vi "calc_VoltageRampWaveform_v0.03.vi"(0 "New input cluster":T1={"Which Position to use for Experiment"=enum."Jumper Safe Position", "Duration (s)"=0.0, "Delay (s)"=0.0, "Ramp Slope (mV/s)"=0.0, "Voltage Start (mV)"=1.0, "Replicates"=1.0, "Voltage End (mV)"=1.0, "Ramp Duration (s)"=0.0, "Vholding (mV)"=0.0, "Valve 1 Position"=2, "Valve 2 Position"=2, "Valve 3 Position"=2, "valve 1 used now?"=TRUE, "valve 2 used now?"=FALSE, "valve 3 used now? "=FALSE, "Maintain Final Voltage until end?"=TRUE, "protocol Preview"=[]} {"Valve 3 Position" min=1 max=8; "Valve 2 Position" min=1 max=8}, 1 "Clear Waveform?":bool, 5 "Old input cluster":T1={"Which Position to use for Experiment"=enum."Jumper Safe Position", "Duration (s)"=0.0, "Delay (s)"=0.0, "Ramp Slope (mV/s)"=0.0, "Voltage Start (mV)"=1.0, "Replicates"=1.0, "Voltage End (mV)"=1.0, "Ramp Duration (s)"=0.0, "Vholding (mV)"=0.0, "Valve 1 Position"=2, "Valve 2 Position"=2, "Valve 3 Position"=2, "valve 1 used now?"=TRUE, "valve 2 used now?"=FALSE, "valve 3 used now? "=FALSE, "Maintain Final Voltage until end?"=TRUE, "protocol Preview"=[]} {"Valve 3 Position" min=1 max=8; "Valve 2 Position" min=1 max=8}, 7 "sample freq":i32=10000, 11 "error in":errorcluster) -> (4 "output cluster":T1={"Which Position to use for Experiment"=enum."Jumper Safe Position", "Duration (s)"=0.0, "Delay (s)"=0.0, "Ramp Slope (mV/s)"=0.0, "Voltage Start (mV)"=1.0, "Replicates"=1.0, "Voltage End (mV)"=1.0, "Ramp Duration (s)"=0.0, "Vholding (mV)"=0.0, "Valve 1 Position"=2, "Valve 2 Position"=2, "Valve 3 Position"=2, "valve 1 used now?"=TRUE, "valve 2 used now?"=FALSE, "valve 3 used now? "=FALSE, "Maintain Final Voltage until end?"=TRUE, "protocol Preview"=[]} {"Valve 3 Position" min=1 max=8; "Valve 2 Position" min=1 max=8}, 15 "error out":errorcluster)   [LabVIEW 2019]
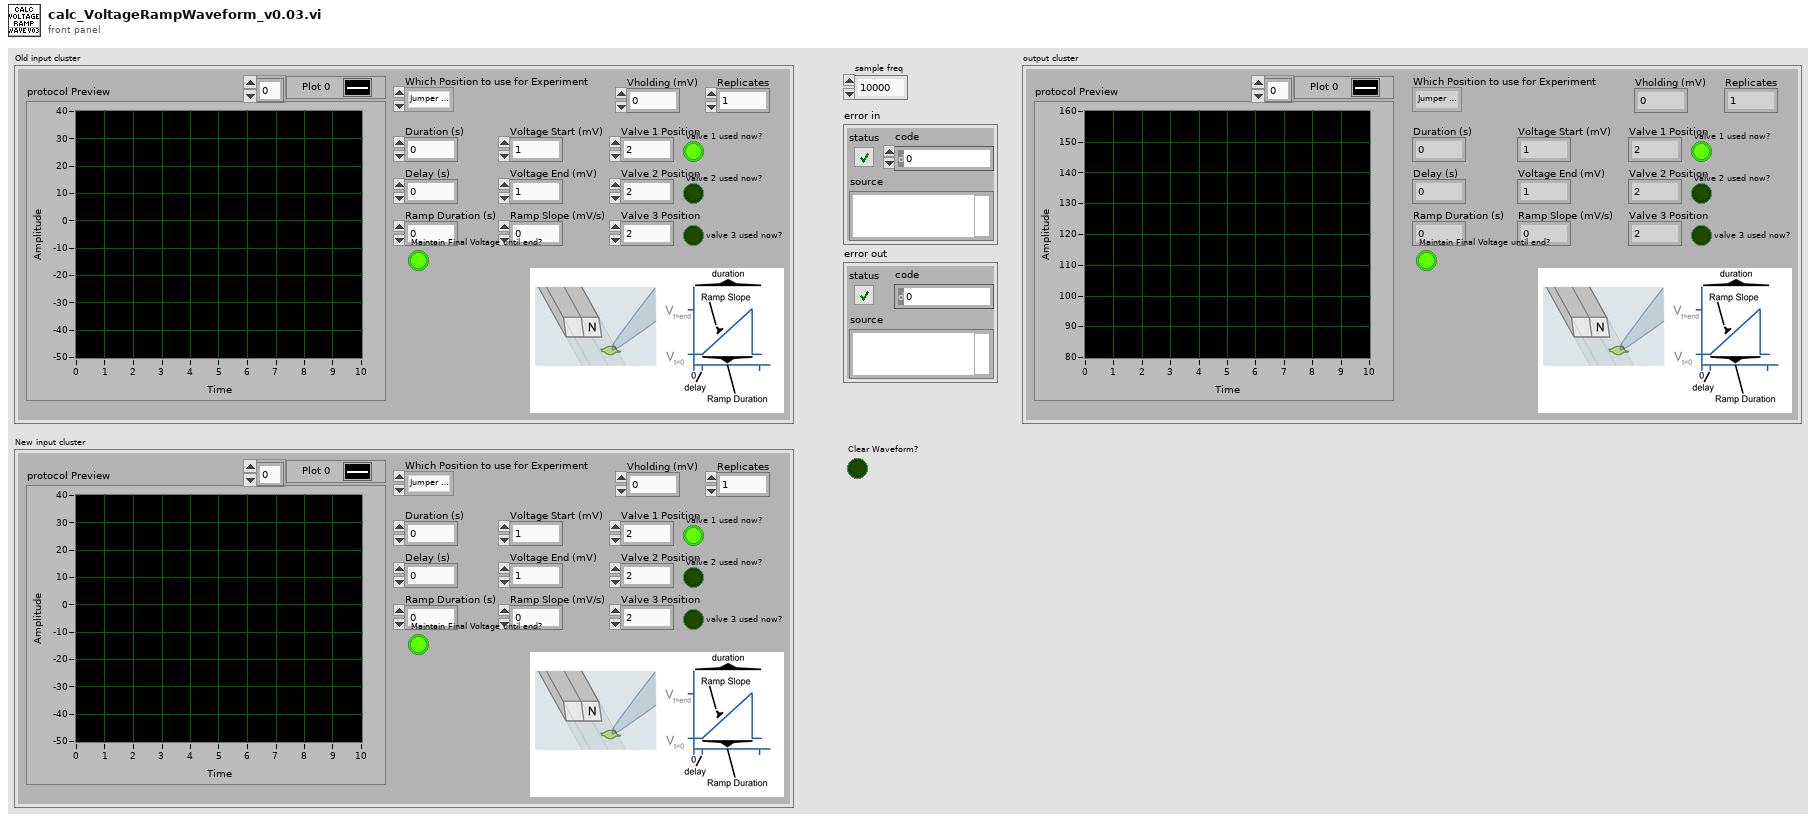
[diagram p1: front panel]
types:
  T1 = cluster{"Which Position to use for Experiment":enum16{"Jumper Safe Position", "Experiment Safe Position", "Jumper Position A", "Jumper Position B", "Jumper Position C", "Jumper Position o-A", "Jumper Position A-o", "Jumper Position A-B", "Jumper Position B-A", "Jumper Position B-C", "Jumper Position C-B", "Jumper Position C-o", "Jumper Position o-C", "Don't Move"}, "Duration (s)":dbl, "Delay (s)":dbl, "Ramp Slope (mV/s)":dbl, "Voltage Start (mV)":dbl, "Replicates":dbl, "Voltage End (mV)":dbl, "Ramp Duration (s)":dbl, "Vholding (mV)":dbl, "Valve 1 Position":i16, "Valve 2 Position":i16, "Valve 3 Position":i16, "valve 1 used now?":bool, "valve 2 used now?":bool, "valve 3 used now? ":bool, "Maintain Final Voltage until end?":bool, "protocol Preview":waveform(dbl)[]}
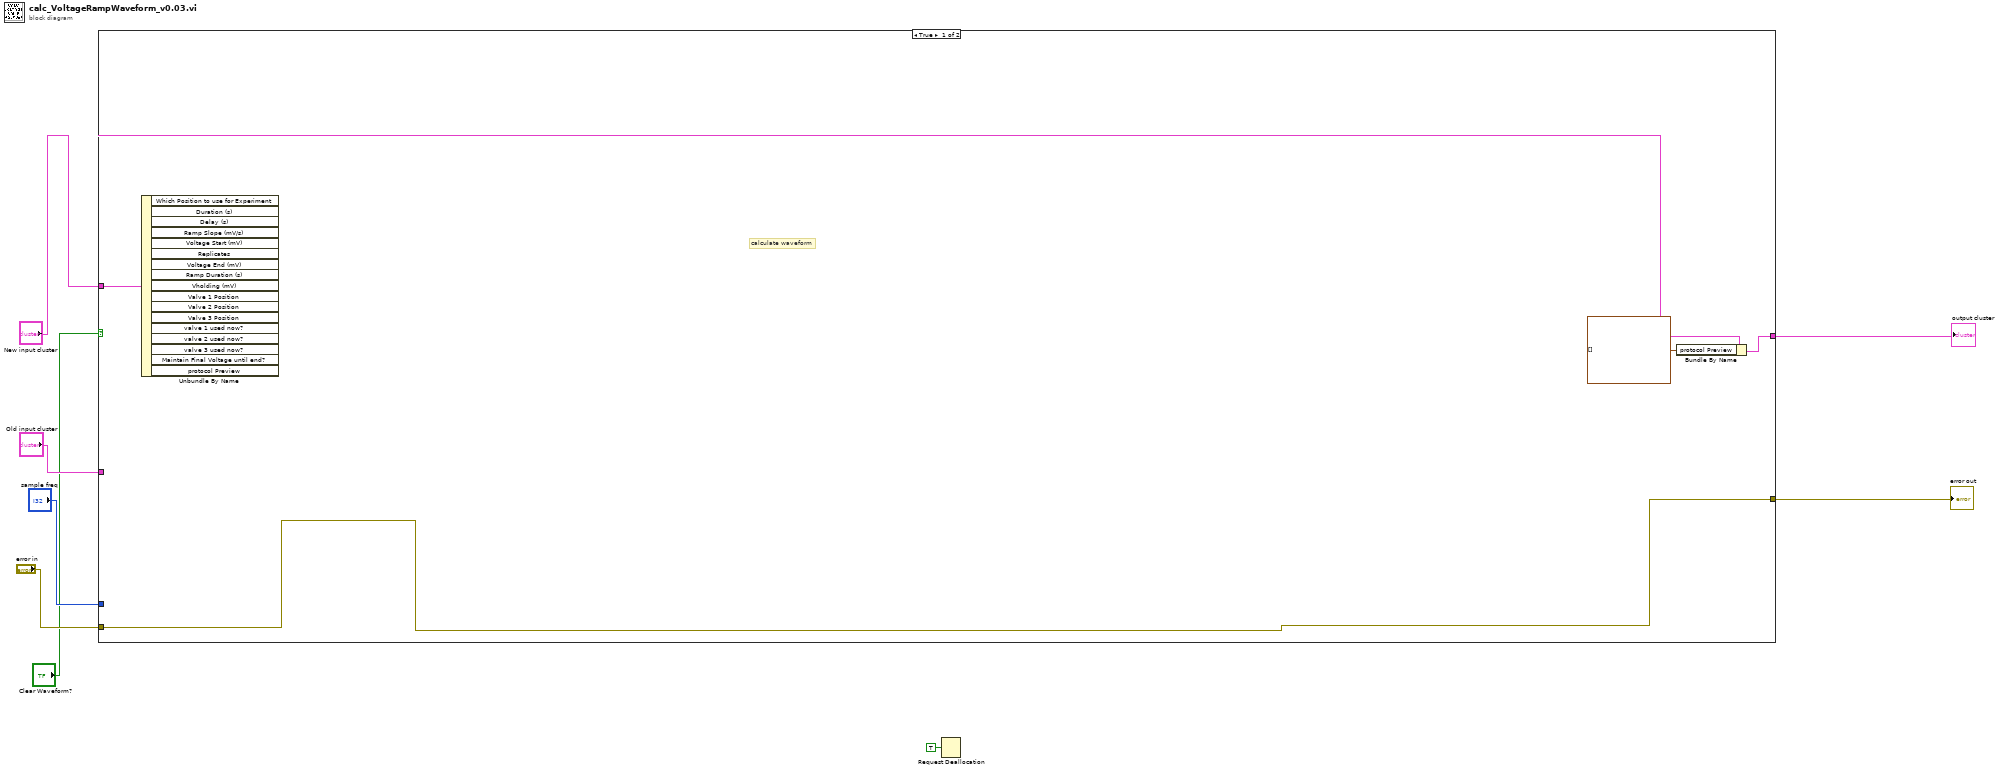
[diagram p0: block diagram]
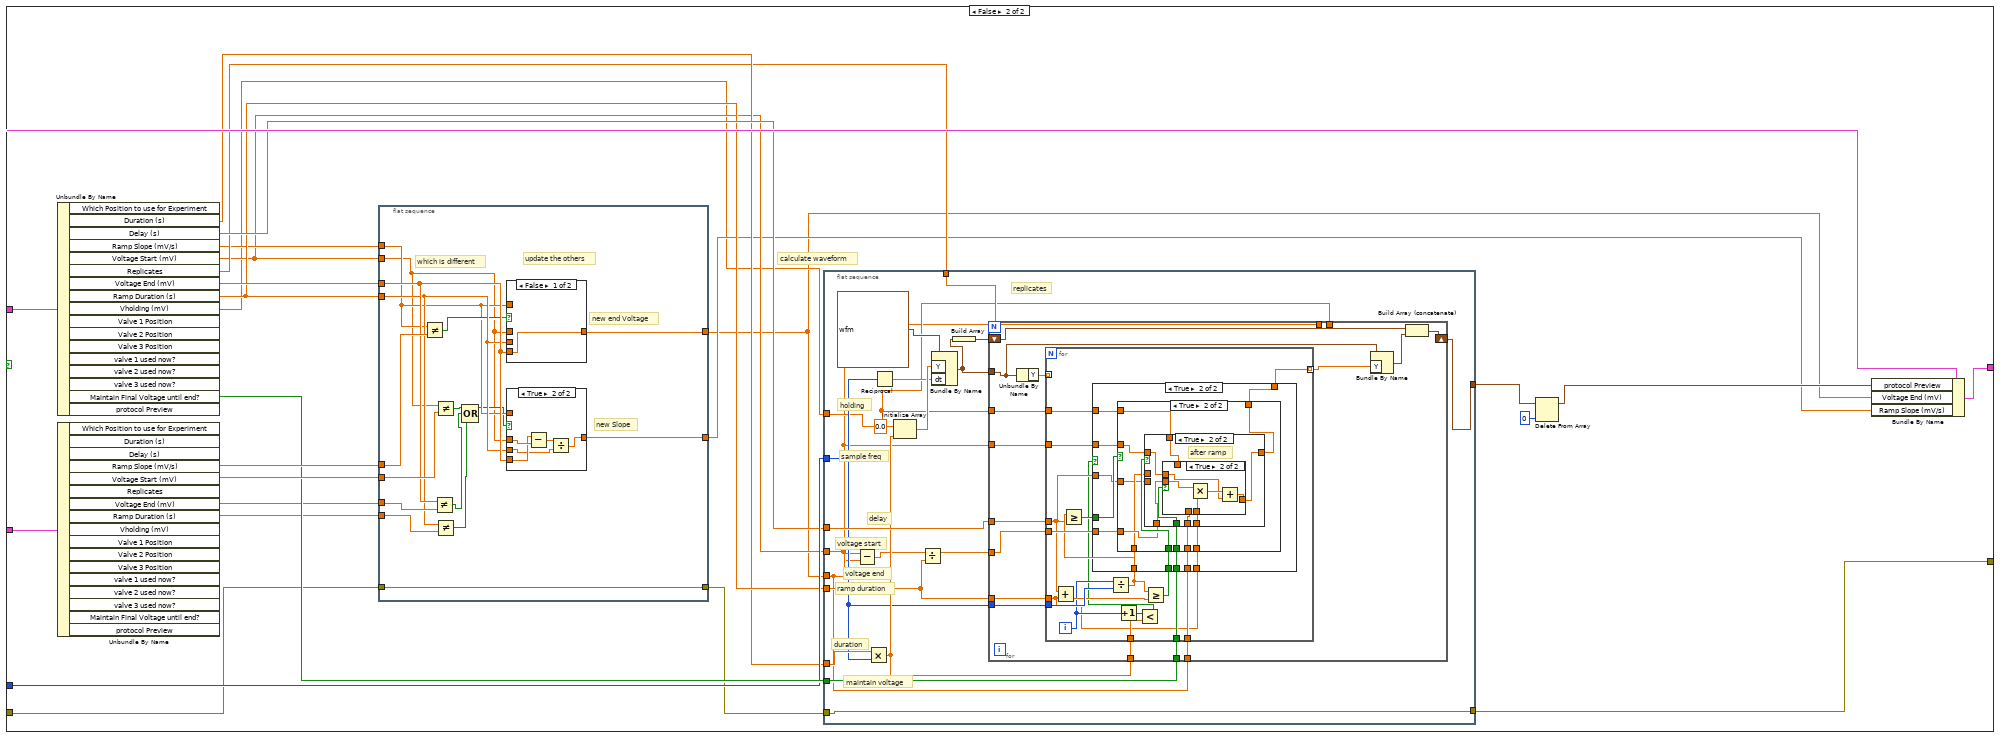
[diagram p2: hidden frame]
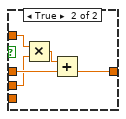
[diagram p4: hidden frame]
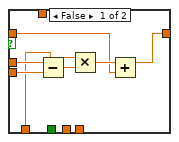
[diagram p7: hidden frame]
diagram:
  n1 = case shown="True" "Clear Waveform?" {
    tunnel: "New input cluster" -> [w12 w37]
    tunnel: [w11 w36] -> w7
    tunnel: "Old input cluster" -> [_ w35]
    tunnel: "sample freq" -> [_ w28]
    tunnel: [w10 w24] -> w4
    tunnel: "error in" -> [w10 w18]
    frame True {
      # "calculate waveform"
      n2 = Unbundle By Name(w12) -> ()  [unwired: 17 out]
      n3 = Bundle By Name(cluster=w12, "protocol Preview"=waveform(dbl)[] []) -> (w11:T1)
    }
    frame False {
      # "calculate waveform"
      n4 = Unbundle By Name(w37) -> ("Duration (s)"=w25:dbl, "Delay (s)"=w27:dbl, "Ramp Slope (mV/s)"=w21:dbl, "Voltage Start (mV)"=w20:dbl, "Replicates"=w23:dbl, "Voltage End (mV)"=w29:dbl, "Ramp Duration (s)"=w26:dbl, "Vholding (mV)"=w17:dbl, "Maintain Final Voltage until end?"=w32:bool)  [unwired: 8 out]
      n5 = Unbundle By Name(w35) -> ("Ramp Slope (mV/s)"=w34:dbl, "Voltage Start (mV)"=w33:dbl, "Voltage End (mV)"=w31:dbl, "Ramp Duration (s)"=w30:dbl)  [unwired: 13 out]
      n6 = flat-sequence {
        tunnel: w34 -> [w53]
        tunnel: w33 -> [w52]
        tunnel: w31 -> [w51]
        tunnel: w30 -> [w50]
        tunnel: w29 -> [w49]
        tunnel: [w48] -> w16
        tunnel: w26 -> [w47]
        tunnel: w21 -> [w44]
        tunnel: w20 -> [w40]
        tunnel: [w39] -> w19
        tunnel: w18 -> [w38]
        tunnel: [w38] -> w13
        frame #0 {
          # "new Slope"
          # "new end Voltage"
          # "update the others"
          # "which is different"
          n7 = Not Equal?(x=w44, y=w53) -> (x != y?=w46:bool)
          n8 = Not Equal?(x=w49, y=w51) -> (x != y?=w42:bool)
          n9 = Not Equal?(x=w40, y=w52) -> (x != y?=w45:bool)
          n10 = Not Equal?(x=w47, y=w50) -> (x != y?=w41:bool)
          n11 = Compound Arithmetic op=OR(w45, w42, w41) -> (w43:bool)
          n12 = case shown="False" w46 {
            tunnel: w44 -> [_ w61]
            tunnel: w49 -> [w60 _]
            tunnel: w40 -> [_ w65]
            tunnel: w47 -> [_ w63]
            tunnel: [w60 w64] -> w48
            frame False {
            }
            frame True {
              n13 = Multiply(x=w61, y=w63) -> (x*y=w62:dbl)
              n14 = Add(x=w62, y=w65) -> (x+y=w64:dbl)
            }
          }
          n15 = case shown="True" w43 {
            tunnel: w44 -> [w54 _]
            tunnel: w49 -> [_ w58]
            tunnel: w40 -> [_ w59]
            tunnel: w47 -> [_ w56]
            tunnel: [w54 w55] -> w39
            frame False {
            }
            frame True {
              n16 = Subtract(x=w58, y=w59) -> (x-y=w57:dbl)
              n17 = Divide(x=w57, y=w56) -> (x/y=w55:dbl)
            }
          }
        }
      }
      n18 = flat-sequence {
        tunnel: w25 -> [w84]
        tunnel: w13 -> [w72]
        tunnel: w27 -> [w79]
        tunnel: [w66] -> _
        tunnel: w23 -> [w85]
        tunnel: w28 -> [w73]
        tunnel: w17 -> [w68]
        tunnel: w16 -> [w69]
        tunnel: w26 -> [w78]
        tunnel: w32 -> [w75]
        tunnel: [w74] -> w14
        tunnel: w20 -> [w66]
        tunnel: [w72] -> w24
        frame #0 {
          # "maintain voltage"
          # "duration"
          # "ramp duration"
          # "voltage end"
          # "voltage start"
          # "delay"
          # "replicates"
          # "sample freq"
          # "holding"
          n19 = Subtract(x=w69, y=w66) -> (x-y=w70:dbl)
          n20 = Multiply(x=w84, y=w73) -> (x*y=w76:dbl)
          n21 = Reciprocal(x=w73) -> (1/x=w77:dbl)
          n22 = Initialize Array(0.0 ("element"), w76) -> (w81:dbl[])
          n23 = Divide(x=w70, y=w78) -> (x/y=w80:dbl)
          n24 = Bundle By Name(cluster=waveform(dbl) {"t0"=timestamp(0 s since 1904-01-01), "dt"=1.0, "Y"=[]} ("signal out"), "Y"=w81, "dt"=w77) -> (w71:waveform(dbl))
          n25 = Build Array(w71) -> (w83:waveform(dbl)[])
          n26 = for {
            N: w85 -> [_]
            shift-right: [w100] -> w74
            shift-left: w83 -> [w99]
            tunnel: w71 -> [w96]
            tunnel: w80 -> [w91]
            tunnel: w73 -> [w95]
            tunnel: w79 -> [w94]
            tunnel: w78 -> [w93]
            tunnel: w66 -> [w92]
            tunnel: w76 -> [w90]
            tunnel: w68 -> [_]
            tunnel: w75 -> [w89]
            tunnel: w66 -> [_]
            tunnel: w68 -> [w88]
            tunnel: w69 -> [w87]
            n27 = Unbundle By Name(w96) -> ("Y"=w97:dbl[])
            n28 = for {
              tunnel: [w101] -> w86 mode=indexing
              tunnel: w97 -> [_] mode=indexing
              tunnel: w95 -> [w117]
              tunnel: w94 -> [w110]
              tunnel: w93 -> [w102]
              tunnel: w92 -> [w114]
              tunnel: w91 -> [w113]
              tunnel: w90 -> [w109]
              tunnel: w89 -> [w105]
              tunnel: w88 -> [w104]
              tunnel: w87 -> [w103]
              i -> [w108]
              n29 = Add(x=w110, y=w102) -> (x+y=w111:dbl)
              n30 = Divide(x=w108, y=w117) -> (x/y=w112:dbl)
              n31 = Greater Or Equal?(x=w112, y=w110) -> (x >= y?=w116:bool)
              n32 = Increment(x=w108) -> (x+1=w106:i32)
              n33 = Less?(x=w106, y=w109) -> (x < y?=w107:bool)
              n34 = Greater Or Equal?(x=w112, y=w111) -> (x >= y?=w115:bool)
              n35 = case shown="True" w107 {
                tunnel: w116 -> [_ w129]
                tunnel: [w118 w128] -> w101
                tunnel: w115 -> [_ w127]
                tunnel: w114 -> [w118 w126]
                tunnel: w113 -> [_ w125]
                tunnel: w112 -> [_ w124]
                tunnel: w110 -> [_ w123]
                tunnel: w105 -> [_ w122]
                tunnel: w104 -> [_ w121]
                tunnel: w103 -> [_ w120]
                tunnel: w102 -> [_ w119]
                frame False {
                  # "last sample"
                }
                frame True {
                  n36 = case shown="True" w129 {
                    tunnel: [w130 w138] -> w128
                    tunnel: w127 -> [_ w140]
                    tunnel: w126 -> [w130 w139]
                    tunnel: w125 -> [_ w137]
                    tunnel: w124 -> [_ w136]
                    tunnel: w123 -> [_ w135]
                    tunnel: w122 -> [_ w134]
                    tunnel: w121 -> [_ w133]
                    tunnel: w120 -> [_ w132]
                    tunnel: w119 -> [_ w131]
                    frame False {
                      # "before delay"
                    }
                    frame True {
                      n37 = case shown="True" w140 {
                        tunnel: w139 -> [w141 w153]
                        tunnel: [w142 w152] -> w138
                        tunnel: w137 -> [w143 w149]
                        tunnel: w136 -> [w146 _]
                        tunnel: w135 -> [w147 _]
                        tunnel: w134 -> [_ w154]
                        tunnel: w133 -> [_ w151]
                        tunnel: w132 -> [_ w150]
                        tunnel: w131 -> [_ w148]
                        frame False {
                          n38 = Subtract(x=w146, y=w147) -> (x-y=w145:dbl)
                          n39 = Multiply(x=w143, y=w145) -> (x*y=w144:dbl)
                          n40 = Add(x=w144, y=w141) -> (x+y=w142:dbl)
                        }
                        frame True {
                          # "after ramp"
                          n41 = case shown="True" w154 {
                            tunnel: w153 -> [w155 w158]
                            tunnel: [w155 w159] -> w152
                            tunnel: w151 -> [_ _]
                            tunnel: w150 -> [_ _]
                            tunnel: w149 -> [_ w157]
                            tunnel: w148 -> [_ w156]
                            frame False {
                            }
                            frame True {
                              n42 = Multiply(x=w157, y=w156) -> (x*y=w160:dbl)
                              n43 = Add(x=w160, y=w158) -> (x+y=w159:dbl)
                            }
                          }
                        }
                      }
                    }
                  }
                }
              }
            }
            n44 = Bundle By Name(cluster=w96, "Y"=w86) -> (w98:waveform(dbl))
            n45 = Build Array (concatenate)(w99, w98) -> (w100:waveform(dbl)[])
          }
        }
      }
      n46 = Delete From Array(array=w14, index=0) -> (array with subset deleted=w22:waveform(dbl)[])  [unwired: 1 in, 1 out]
      n47 = Bundle By Name(cluster=w37, "protocol Preview"=w22, "Voltage End (mV)"=w16, "Ramp Slope (mV/s)"=w19) -> (w36:T1)
    }
  }
  "output cluster" <- w7
  "error out" <- w4
  n48 = Request Deallocation(TRUE ("flag")) -> ()
